vi "Master VI.vi"() -> ()   [LabVIEW 2020]
uses:
  <vilib>/Platform/browser.llb/Open URL in Default Browser (string).vi
  MainVIs.lvlib
  AnalysisSupport.lvlib
  <resource>/objmgr/daqmx.rc
panel:
  in  "Stenosis Testing":bool
  in  "Fix LVM Button":bool
  in  "Extract F0":bool
  in  "Extract Button":bool
  in  "Report Error or Request Change":bool
  in  "SPL":bool
  in  "Calibration":bool
  in  "Analysis":bool
  in  "Clipper":bool
  in  "Singing Helmet":bool
  in  "Redirect":bool
  in  "Complete":bool
  in  "Exit Button":bool
  in  "Incomplete":bool
  # "Select a Program"
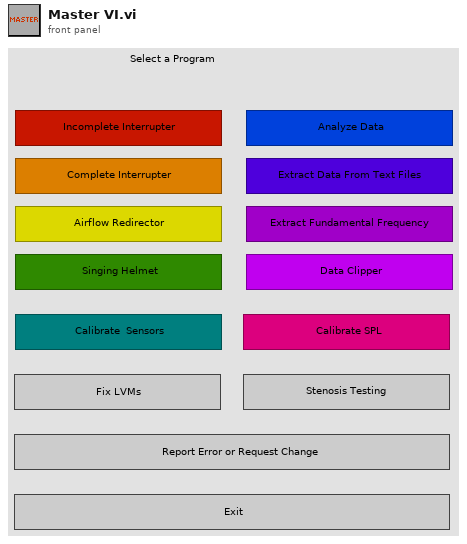
[diagram p1: front panel]
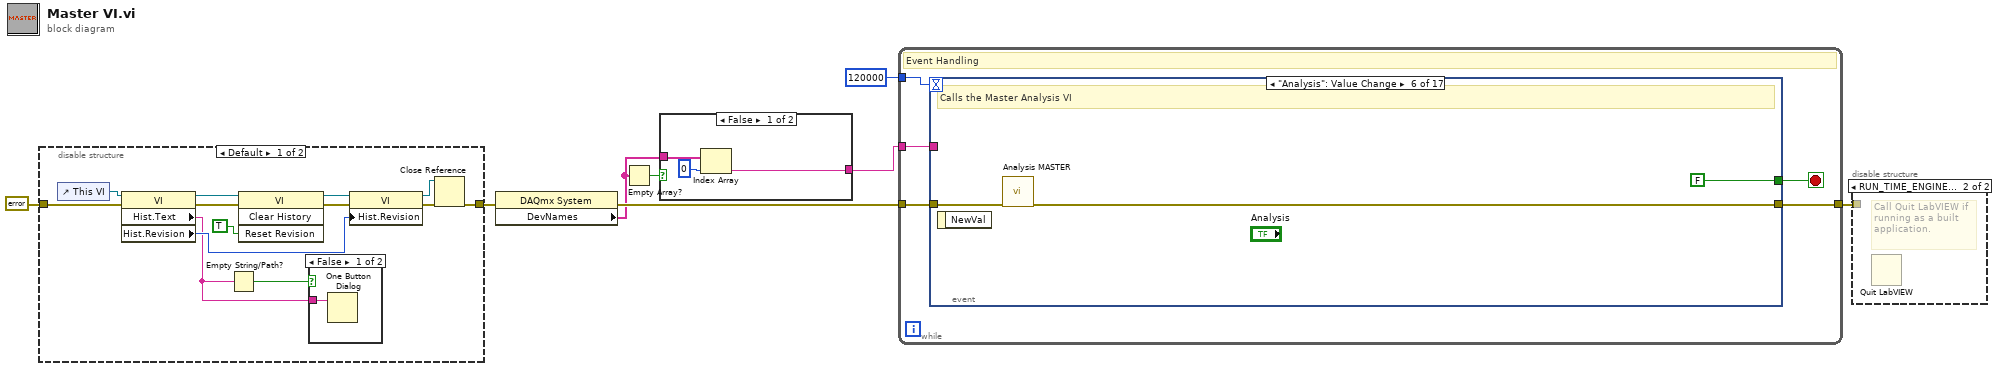
[diagram p0: block diagram]
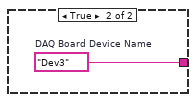
[diagram p2: hidden frame]
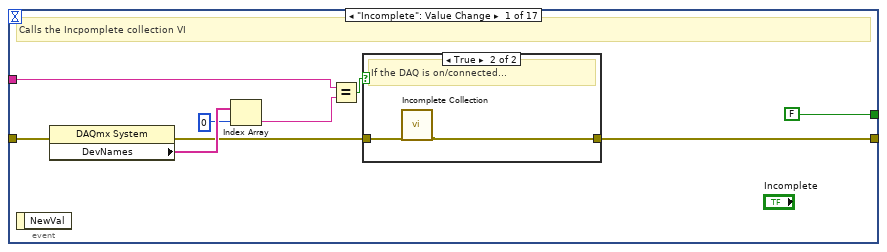
[diagram p6: hidden frame]
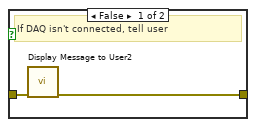
[diagram p7: hidden frame]
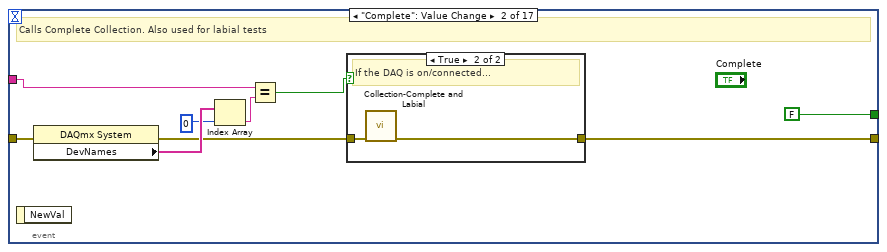
[diagram p8: hidden frame]
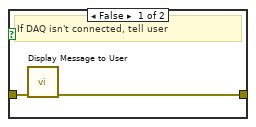
[diagram p9: hidden frame]
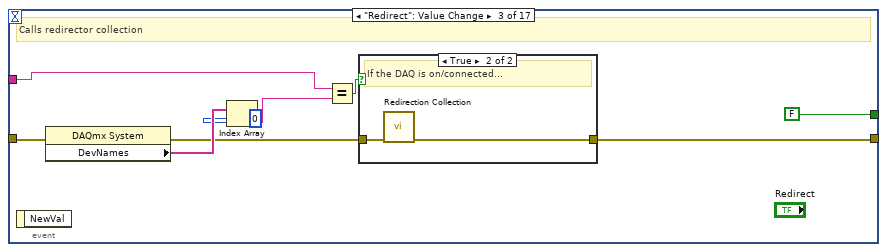
[diagram p10: hidden frame]
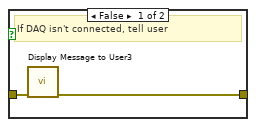
[diagram p11: hidden frame]
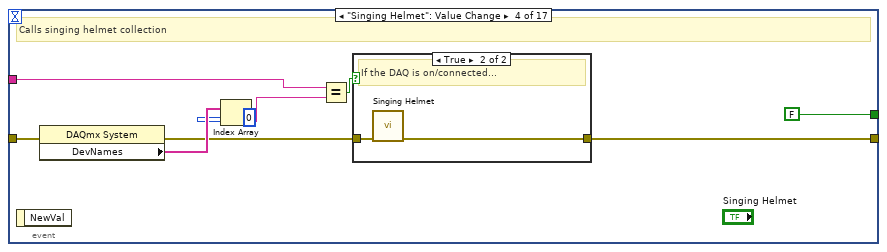
[diagram p12: hidden frame]
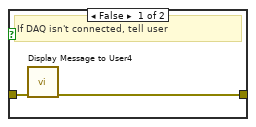
[diagram p13: hidden frame]
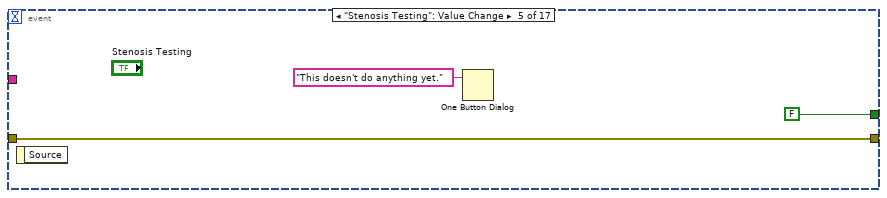
[diagram p14: hidden frame]
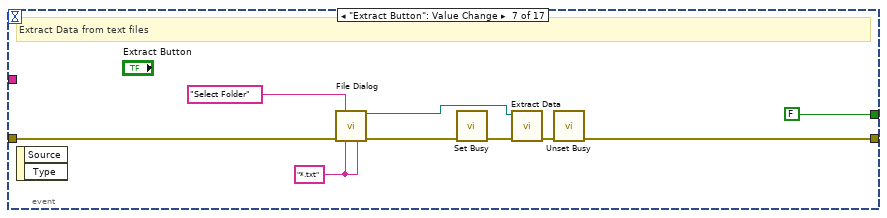
[diagram p15: hidden frame]
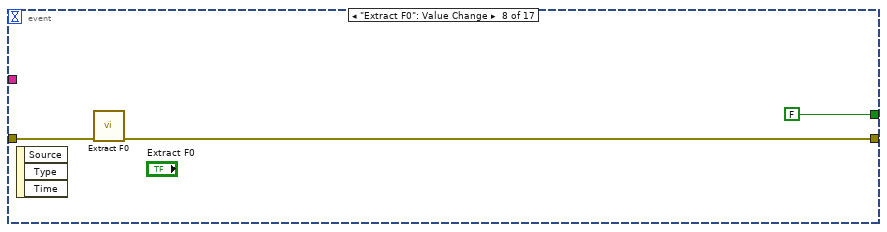
[diagram p16: hidden frame]
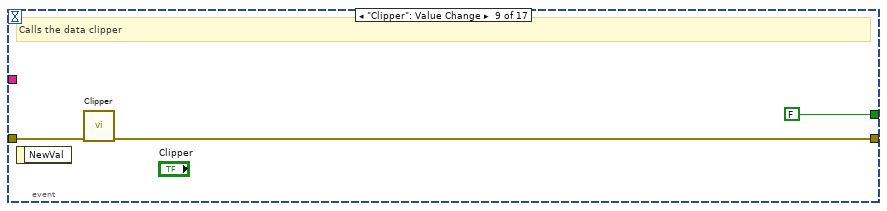
[diagram p17: hidden frame]
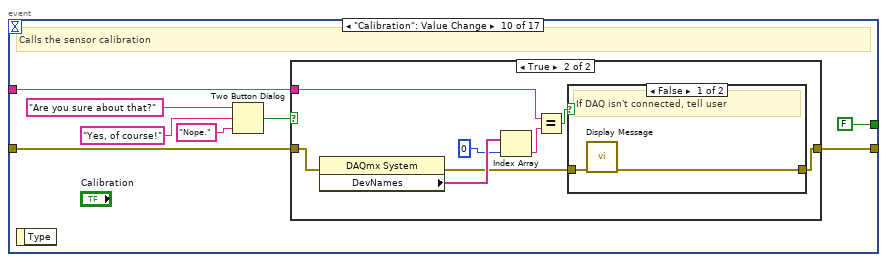
[diagram p18: hidden frame]
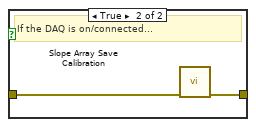
[diagram p20: hidden frame]
diagram:
  n1 = disable-structure shown="Default" {
    disable-tunnel: errorcluster {"status"=FALSE, "code"=0, "source"=""} ("error constant") -> [w10 w23]
    disable-tunnel: [w9 w23] -> w5
    frame condition #0 (active) {
      n2 = control-ref of="This VI"() -> (w14:refnum<vi>)
      n3 = property class="VI"(reference=w14, error in=w10) -> (reference out=w12:refnum<vi>, error out=w13:errorcluster, "Hist.Text"=w15:string, "Hist.Revision"=w21:u32)
      n4 = Empty String/Path?(string/path=w15) -> (empty?=w16:bool)
      n5 = invoke class="VI" method="Clear History"(reference=w12, error in=w13, "Reset Revision"=TRUE) -> (reference out=w17:refnum<vi>, error out=w18:errorcluster)  [unwired: 1 in, 2 out]
      n6 = case shown="False" w16 {
        tunnel: w15 -> [w22 _]
        frame False {
          n7 = One Button Dialog(message=w22) -> ()  [unwired: 1 in, 1 out]
        }
        frame True {
        }
      }
      n8 = property class="VI"(reference=w17, error in=w18, "Hist.Revision"=w21) -> (reference out=w19:refnum<vi>, error out=w20:errorcluster)
      n9 = Close Reference(reference=w19, error in (no error)=w20) -> (error out=w9:errorcluster)
    }
    frame condition #1 {
    }
  }
  n10 = property class="DAQmx System"(error in=w5) -> (error out=w4:errorcluster, "DevNames"=w1:tag[])  [unwired: 1 in, 1 out]
  n11 = Empty Array?(array=w1) -> (empty?=w3:bool)
  n12 = case shown="False" w3 {
    tunnel: [w24 w27] -> w2
    tunnel: w1 -> [w25 _]
    frame False {
      n13 = Index Array(array=w25, index=0) -> (element=w24:tag)
    }
    frame True {
      w27 = tag "Dev3"  # DAQ Board Device Name
    }
  }
  n14 = while {
    tunnel: [w31] -> w8
    tunnel: w4 -> [w30]
    tunnel: 120000 -> [w29]
    tunnel: w2 -> [w28]
    stop <- w32 stop-if-true
    # "Event Handling"
    n15 = event shown="[5] \"Analysis\": Value Change" {
      selector: _ -> [_ _ _ _ _ _ _ _ _ _ _ _ _ _ _ _ _]
      dyn-events: _ -> [_ _ _ _ _ _ _ _ _ _ _ _ _ _ _ _ _]
      timeout: w29 -> [_ _ _ _ _ _ _ _ _ _ _ _ _ _ _ _ _]
      tunnel: [FALSE FALSE FALSE FALSE FALSE FALSE FALSE FALSE FALSE FALSE FALSE FALSE FALSE TRUE w153 TRUE TRUE] -> w32
      tunnel: [w34 w48 w60 w73 w87 w89 w92 w101 w104 w112 w132 w139 w144 w151 w155 w157 w160] -> w31
      tunnel: w30 -> [w35 w47 w61 w74 w87 w90 w96 w102 w105 w113 w133 w140 w143 w151 w156 w157 w160]
      tunnel: w28 -> [w33 w46 w59 w72 _ _ _ _ _ w106 _ _ _ _ _ _ _]
      event "Incomplete": Value Change {
        # "Calls the Incpomplete collection VI"
        n16 = event-data() -> ()  [unwired: 1 in, 1 out]
        n17 = property class="DAQmx System"(error in=w35) -> (error out=w39:errorcluster, "DevNames"=w40:tag[])  [unwired: 1 in, 1 out]
        n18 = Index Array(array=w40, index=0) -> (element=w38:tag)
        n19 = Equal?(x=w33, y=w38) -> (x = y?=w37:bool)
        n20 = case shown="True" w37 {
          tunnel: w39 -> [w43 w45]
          tunnel: [w42 w44] -> w34
          frame False {
            # "If DAQ isn't connected, tell user"
            n21 = call "Display Message to User2"("error in (no error)"=w43) -> ("error out"=w42:errorcluster)  [unwired: 9 in, 1 out]
          }
          frame True {
            # "If the DAQ is on/connected..."
            n22 = call "Incomplete Collection.vi"("error in (no error)"=w45) -> ("error out"=w44:errorcluster)  [unwired: 10 in]
          }
        }
      }
      event "Complete": Value Change {
        # "Calls Complete Collection. Also used for labial tests"
        n23 = event-data() -> ()  [unwired: 1 in, 1 out]
        n24 = property class="DAQmx System"(error in=w47) -> (error out=w52:errorcluster, "DevNames"=w53:tag[])  [unwired: 1 in, 1 out]
        n25 = Index Array(array=w53, index=0) -> (element=w51:tag)
        n26 = Equal?(x=w46, y=w51) -> (x = y?=w50:bool)
        n27 = case shown="True" w50 {
          tunnel: w52 -> [w56 w58]
          tunnel: [w55 w57] -> w48
          frame False {
            # "If DAQ isn't connected, tell user"
            n28 = call "Display Message to User"("error in (no error)"=w56) -> ("error out"=w55:errorcluster)  [unwired: 9 in, 1 out]
          }
          frame True {
            # "If the DAQ is on/connected..."
            n29 = call "Collection-Complete and Labial.vi"("error in"=w58) -> ("error out"=w57:errorcluster)  [unwired: 10 in]
          }
        }
      }
      event "Redirect": Value Change {
        # "Calls redirector collection"
        n30 = event-data() -> ()  [unwired: 1 in, 1 out]
        n31 = property class="DAQmx System"(error in=w61) -> (error out=w65:errorcluster, "DevNames"=w66:tag[])  [unwired: 1 in, 1 out]
        n32 = Index Array(array=w66, index=0) -> (element=w64:tag)
        n33 = Equal?(x=w59, y=w64) -> (x = y?=w63:bool)
        n34 = case shown="True" w63 {
          tunnel: w65 -> [w69 w70]
          tunnel: [w68 w71] -> w60
          frame False {
            # "If DAQ isn't connected, tell user"
            n35 = call "Display Message to User3"("error in (no error)"=w69) -> ("error out"=w68:errorcluster)  [unwired: 9 in, 1 out]
          }
          frame True {
            # "If the DAQ is on/connected..."
            n36 = call "Redirection Collection.vi"("error in"=w70) -> ("error out"=w71:errorcluster)  [unwired: 10 in]
          }
        }
      }
      event "Singing Helmet": Value Change {
        # "Calls singing helmet collection"
        n37 = event-data() -> ()  [unwired: 1 in, 1 out]
        n38 = property class="DAQmx System"(error in=w74) -> (error out=w78:errorcluster, "DevNames"=w79:tag[])  [unwired: 1 in, 1 out]
        n39 = Index Array(array=w79, index=0) -> (element=w77:tag)
        n40 = Equal?(x=w72, y=w77) -> (x = y?=w76:bool)
        n41 = case shown="True" w76 {
          tunnel: w78 -> [w82 w84]
          tunnel: [w81 w83] -> w73
          frame False {
            # "If DAQ isn't connected, tell user"
            n42 = call "Display Message to User4"("error in (no error)"=w82) -> ("error out"=w81:errorcluster)  [unwired: 9 in, 1 out]
          }
          frame True {
            # "If the DAQ is on/connected..."
            n43 = call "Singing Helmet.vi"("error in (no error)"=w84) -> ("error out"=w83:errorcluster)  [unwired: 10 in]
          }
        }
      }
      event "Stenosis Testing": Value Change {
        n44 = event-data() -> ()  [unwired: 1 in, 1 out]
        n45 = One Button Dialog(message="This doesn't do anything yet.") -> ()  [unwired: 1 in, 1 out]
      }
      event "Analysis": Value Change {
        # "Calls the Master Analysis VI"
        n46 = event-data() -> ()  [unwired: 1 in, 1 out]
        n47 = call "Analysis MASTER.vi"("Error In"=w90) -> ("Error Out"=w89:errorcluster)  [unwired: 10 in]
      }
      event "Extract Button": Value Change {
        w98 = "*.txt" ("pattern label")
        # "Extract Data from text files"
        n48 = event-data() -> ()  [unwired: 1 in, 2 out]
        n49 = call "File Dialog"("prompt"="Select Folder", "error in"=w96, "pattern (all files)"=w98, "pattern label"=w98) -> ("selected path"=w97:path, "error out"=w95:errorcluster)  [unwired: 8 in, 2 out]
        n50 = call <vilib>:"Set Busy.vi"("error in (no error)"=w95) -> ("error out"=w94:errorcluster)  [unwired: 9 in, 1 out]
        n51 = call "Extract Data.vi"("Error In"=w94, "Folder Path"=w97) -> ("Error Out"=w93:errorcluster)  [unwired: 9 in]
        n52 = call <vilib>:"Unset Busy.vi"("error in (no error)"=w93) -> ("error out"=w92:errorcluster)  [unwired: 10 in]
      }
      event "Extract F0": Value Change {
        n53 = event-data() -> ()  [unwired: 1 in, 3 out]
        n54 = call "Extract F0.vi"("Error In"=w102) -> ("Error Out"=w101:errorcluster)  [unwired: 10 in]
      }
      event "Clipper": Value Change {
        # "Calls the data clipper"
        n55 = event-data() -> ()  [unwired: 1 in, 1 out]
        n56 = call "Clipper.vi"("error in (no error)"=w105) -> ("error out"=w104:errorcluster)  [unwired: 10 in]
      }
      event "Calibration": Value Change {
        # "Calls the sensor calibration"
        n57 = event-data() -> ()  [unwired: 1 in, 1 out]
        n58 = Two Button Dialog(message="Are you sure about that?", 1:"Nope." ("F button name (\"Cancel\")"), 2:"Yes, of course!" ("T button name (\"OK\")")) -> (T button?=w108:bool)
        n59 = case shown="True" w108 {
          tunnel: w113 -> [w114 w117]
          tunnel: [w114 w116] -> w112
          tunnel: w106 -> [_ w115]
          frame False {
          }
          frame True {
            n60 = property class="DAQmx System"(error in=w117) -> (error out=w121:errorcluster, "DevNames"=w122:tag[])  [unwired: 1 in, 1 out]
            n61 = Index Array(array=w122, index=0) -> (element=w120:tag)
            n62 = Equal?(x=w115, y=w120) -> (x = y?=w119:bool)
            n63 = case shown="False" w119 {
              tunnel: w121 -> [w124 w126]
              tunnel: [w123 w125] -> w116
              frame False {
                # "If DAQ isn't connected, tell user"
                n64 = call "Display Message"("error in (no error)"=w124) -> ("error out"=w123:errorcluster)  [unwired: 9 in, 1 out]
              }
              frame True {
                # "If the DAQ is on/connected..."
                n65 = call "Slope Array Save Calibration.vi"("Error In"=w126) -> ("Error Out"=w125:errorcluster)  [unwired: 11 in, 3 out]
              }
            }
          }
        }
      }
      event "SPL": Value Change {
        (unwired) "C:\\Program Files (x86)\\Audacity\\audacity.exe" ("command line")
        # "Calls the SPL gain estimator"
        n66 = event-data() -> ()  [unwired: 1 in, 2 out]
        n67 = Two Button Dialog(message="Are you sure about that?", 1:"Nope." ("F button name (\"Cancel\")"), 2:"Yes, of course!" ("T button name (\"OK\")")) -> (T button?=w128:bool)
        n68 = case shown="True" w128 {
          tunnel: w133 -> [w134 w136]
          tunnel: [w134 w135] -> w132
          frame False {
          }
          frame True {
            n69 = call "Gain Estimator.vi"("error in (no error)"=w136) -> ("Error Out"=w135:errorcluster)  [unwired: 8 in, 2 out]
          }
        }
      }
      event "Report Error or Request Change": Value Change {
        n70 = event-data() -> ()  [unwired: 1 in, 2 out]
        n71 = call-poly <vilib>:"Open URL in Default Browser.vi"("error in (no error)"=w140, "URL"="https://goo.gl/forms/o6MZTBsEczWoqA8r1") -> ("error out"=w139:errorcluster)  [unwired: 4 in, 1 out]
      }
      event "Fix LVM Button": Value Change {
        # "Runs the LVM Fixer"
        n72 = event-data() -> ()  [unwired: 1 in, 3 out]
        n73 = call "File Dialog - Fixer"("error in"=w143) -> ("selected path"=w146:path, "cancelled"=w142:bool, "error out"=w145:errorcluster)  [unwired: 11 in, 1 out]
        n74 = case shown="False" w142 {
          tunnel: w146 -> [w149 _]
          tunnel: w145 -> [w148 w150]
          tunnel: [w147 w150] -> w144
          frame False {
            n75 = call "Main.vi"("Error In"=w148, "Folder"=w149) -> ("Error Out"=w147:errorcluster)  [unwired: 9 in]
          }
          frame True {
          }
        }
      }
      event "Exit Button": Value Change {
        # "Exits the VI"
        n76 = event-data() -> ()  [unwired: 1 in, 1 out]
      }
      event Timeout {
        n77 = event-data() -> ()  [unwired: 1 in, 3 out]
        n78 = call "Timeout Check.vi"("Error In"=w156) -> ("Error Out"=w155:errorcluster, "Still there?"=w154:bool)  [unwired: 9 in]
        n79 = Not(x=w154) -> (.not. x?=w153:bool)
      }
      event Application Instance Close {
        # "The user has closed the app"
        n80 = event-data() -> ()  [unwired: 1 in, 1 out]
      }
      event Panel Close? {
        # "the panel has been closed"
        n81 = event-data() -> ()  [unwired: 1 in, 1 out]
        n82 = event-data() -> ()  [unwired: 2 in, 1 out]
      }
    }
  }
  n83 = disable-structure shown="RUN_TIME_ENGINE==True" {
    disable-tunnel: w8 -> [_ _]
    frame condition #0 (active) {
    }
    frame condition #1 {
      # "Call Quit LabVIEW if running as a built application."
      n84 = Quit LabVIEW() -> ()  [unwired: 1 in]
    }
  }
